vi "Select Path.vi"(8 "error in (no error)":errorcluster, 10 "File Path":path, 11 "[V] Main UI in":refnum<class "[V] Main UI.lvclass">) -> (0 "error out":errorcluster, 3 "[V] Main UI out":refnum<class "[V] Main UI.lvclass">)   [LabVIEW 2020, in "[V] Main UI.lvlib" / "[V] Main UI.lvclass"]
uses:
  [V] Main UI.lvclass
  Depden On/MVVM Framework/MVVM Abstruct View/MVVM Abstruct View/MVVM Abstruct View.lvclass/MVVM Abstruct View.ctl
  Models/Data Loader/Data Load Interface/Data Load Interface Messages/Select File Msg/Select File Msg.lvclass/Select File Msg.ctl
  <vilib>/ActorFramework/Message Enqueuer/Message Enqueuer.lvclass/Message Enqueuer.ctl
  Depden On/MVVM Framework/MVVM Abstruct View/MVVM Abstruct View/Accessor/Read ActorMap-Models.vi
  <vilib>/ActorFramework/Message Enqueuer/Enqueue.vi
  Models/Data Loader/Data Load Interface/Data Load Interface Messages/Select File Msg/Select File Msg.lvclass
  C:/Program Files (x86)/National Instruments/LabVIEW 2020/vi.lib/ActorFramework/Message/Message.lvclass
  <vilib>/ActorFramework/Message Priority Queue/Priority Enqueue.vi
  Depden On/ActorMap/ActorMap.lvclass
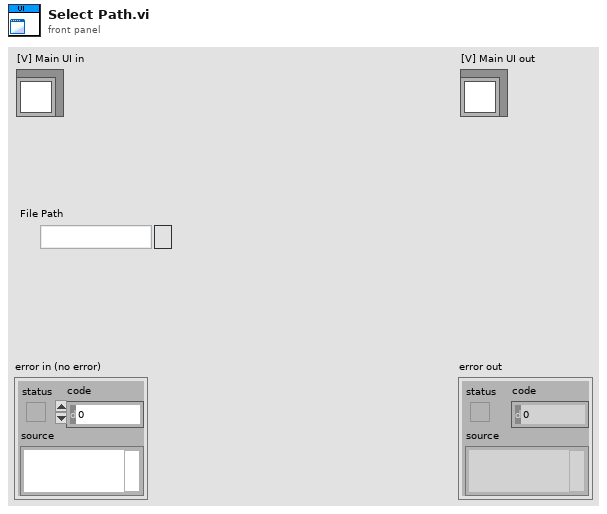
[diagram p1: front panel]
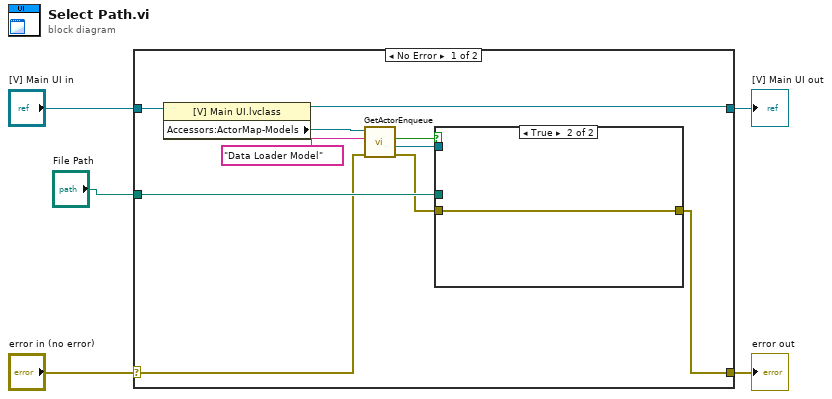
[diagram p0: block diagram]
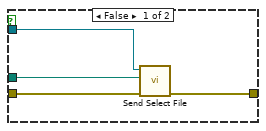
[diagram p2: hidden frame]
diagram:
  n1 = case shown="No Error" "error in (no error)" {
    selector: "error in (no error)" -> [w6 w22]
    tunnel: [w7 w22] -> w4
    tunnel: [w14 w21] -> w2
    tunnel: "[V] Main UI in" -> [w15 w21]
    tunnel: "File Path" -> [w9 _]
    frame No Error {
      n2 = property class="[V] Main UI.lvclass"(reference=w15) -> (reference out=w14:refnum<class "[V] Main UI.lvclass">, "Accessors:ActorMap-Models"=w13:refnum<class "ActorMap.lvclass">)  [unwired: 1 in, 1 out]
      n3 = call "GetActorEnqueue.vi"("error in (no error)"=w6, "name"="Data Loader Model", "ActorMap in"=w13) -> ("error out"=w8:errorcluster, "Enqueue"=w10:refnum<class "Message Enqueuer.lvclass">, "key not found?"=w11:bool)  [unwired: 5 in, 1 out]
      n4 = case shown="True" w11 {
        tunnel: w10 -> [w19 _]
        tunnel: w9 -> [w18 _]
        tunnel: w8 -> [w17 w20]
        tunnel: [w16 w20] -> w7
        frame False {
          n5 = call "Send Select File.vi"("error in (no error)"=w17, "File Path"=w18, "Message Enqueuer"=w19) -> ("error out"=w16:errorcluster)  [unwired: 7 in, 1 out]
        }
        frame True {
        }
      }
    }
    frame Error {
    }
  }
  "error out" <- w4
  "[V] Main UI out" <- w2
